vi "ReadExperimentFile.vi"(10 "BaseSearchPath":path, 11 "ScriptFile":path) -> (0 "Working Directory":path, 2 "FilePath":path, 3 "String":string)   [LabVIEW 2017]
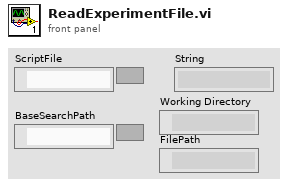
[diagram p1: front panel]
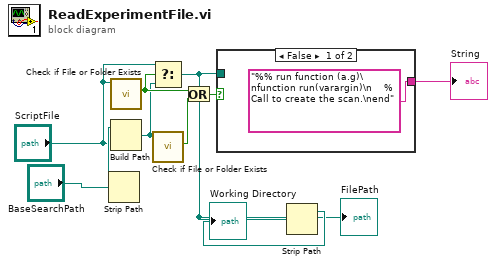
[diagram p0: block diagram]
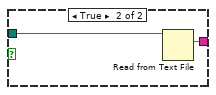
[diagram p2: hidden frame]
diagram:
  n1 = Strip Path(path="BaseSearchPath") -> (stripped path=w10:path)  [unwired: 1 out]
  n2 = call <vilib>:"Check if File or Folder Exists.vi"("path"="ScriptFile") -> ("file or folder exists?"=w7:bool)  [unwired: 8 in, 2 out]
  n3 = Build Path(base path=w10, name or relative path="ScriptFile") -> (appended path=w4:path)
  n4 = Select(t="ScriptFile", s=w7, f=w4) -> (s? t:f=w1:path)
  "FilePath" <- w1
  n5 = call <vilib>:"Check if File or Folder Exists.vi"("path"=w4) -> ("file or folder exists?"=w8:bool)  [unwired: 8 in, 2 out]
  n6 = Or(x=w7, y=w8) -> (x .or. y?=w6:bool)
  n7 = case shown="False" w6 {
    tunnel: w1 -> [_ w13]
    tunnel: ["%% run function (a.g)\nfunction run(varargin)\n    % Call to create the scan.\nend" w12] -> w3
    frame False {
    }
    frame True {
      n8 = Read from Text File(file (use dialog)=w13) -> (text=w12:string)  [unwired: 3 in, 3 out]
    }
  }
  "String" <- w3
  n9 = Strip Path(path=w1) -> (stripped path=→"Working Directory":path)  [unwired: 1 out]
